vi "get_setting.vi"(7 "settings path":path=path "D:/Scripts/AId_SPM_labview/Nanonis Server", 8 "error in (no error)":errorcluster, 9 "section":string="Settings", 10 "FirstRun":bool, 11 "key":string) -> (0 "error out":errorcluster, 1 "output 2":dbl, 2 "output 1":dbl, 3 "value":string="Loaded from:C:\\Users\\cornelik\\AId_SPM_labview\\Nanonis Server\\AId_SPM_server.ini", 4 "Boolean":bool)   [LabVIEW 2019]
uses:
  <vilib>/Utility/config.llb/Read Key (String).vi
  <vilib>/Utility/config.llb/NI_LVConfig.lvlib
panel:
  out "keys":string[][](array[string])
  out "values":string[][](array[string])
  out "sections":string[](array[string])
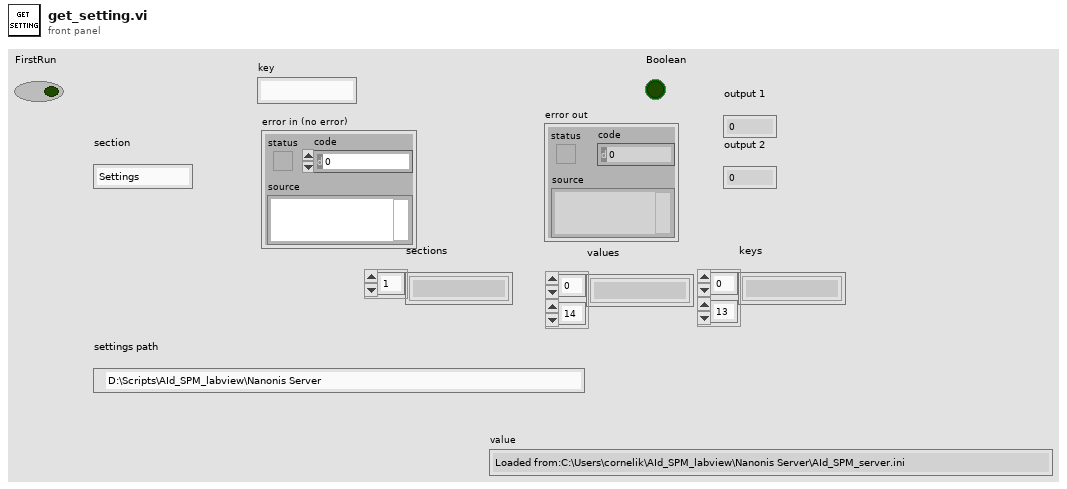
[diagram p1: front panel]
types:
  T1 = typedef "NI_LVConfig.lvlib/Config Data RefNum.ctl" = refnum<k1>
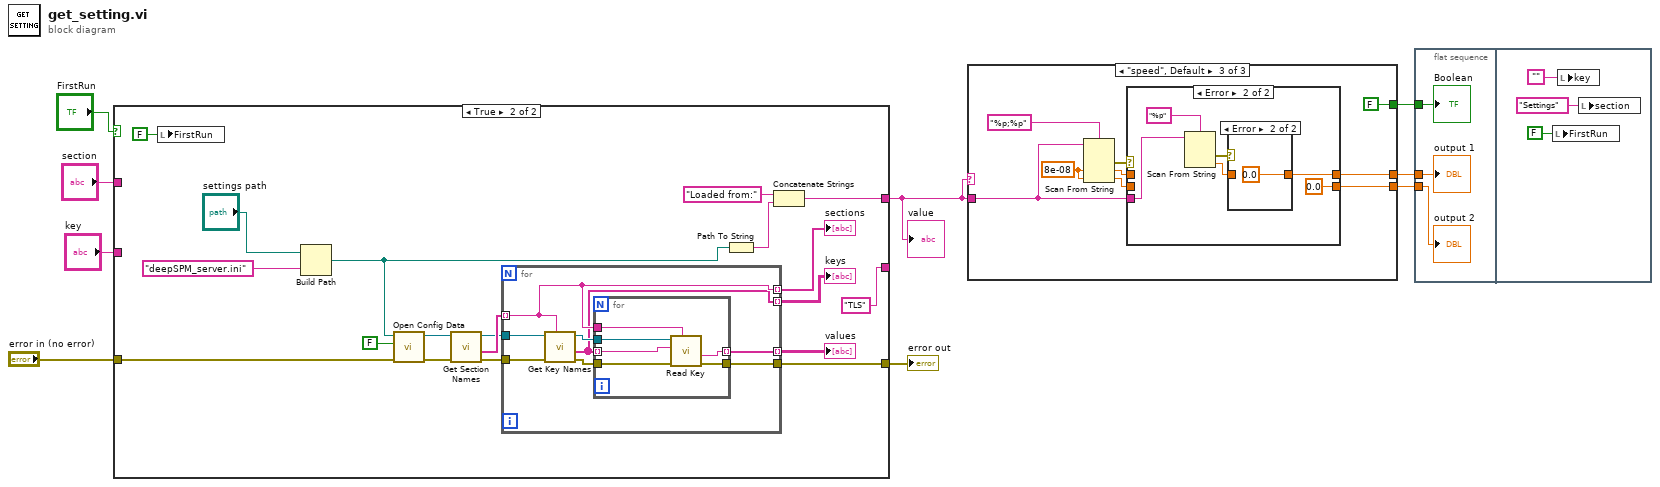
[diagram p0: block diagram]
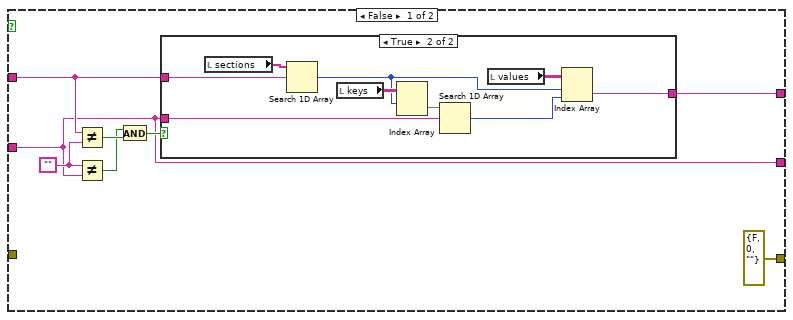
[diagram p2: hidden frame]
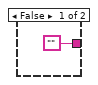
[diagram p3: hidden frame]
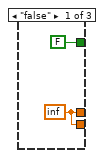
[diagram p4: hidden frame]
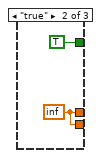
[diagram p5: hidden frame]
diagram:
  n1 = case shown="True" "FirstRun" {
    tunnel: "section" -> [w12 _]
    tunnel: [w17 w32] -> w1
    tunnel: "key" -> [w10 _]
    tunnel: "error in (no error)" -> [_ w35]
    tunnel: [errorcluster {"status"=FALSE, "code"=0, "source"=""} ("error out") w34] -> w4
    tunnel: [w10 "TLS" ("key")] -> _
    frame False {
      w11 = ""
      n2 = Not Equal?(x=w12, y=w11) -> (x != y?=w15:bool)
      n3 = Not Equal?(x=w11, y=w10) -> (x != y?=w13:bool)
      n4 = And(x=w13, y=w15) -> (x .and. y?=w14:bool)
      n5 = case shown="True" w14 {
        tunnel: w12 -> [_ w26]
        tunnel: w10 -> [_ w23]
        tunnel: ["" w20] -> w17
        frame False {
        }
        frame True {
          n6 = local read "sections"() -> (w27:string[])
          n7 = Search 1D Array(1D array=w27, element=w26) -> (index of element=w19:i32)  [unwired: 1 in]
          n8 = local read "keys"() -> (w25:string[][])
          n9 = Index Array(array=w25, index (row)=w19) -> (element=w24:string[])  [unwired: 1 in]
          n10 = Search 1D Array(1D array=w24, element=w23) -> (index of element=w21:i32)  [unwired: 1 in]
          n11 = local read "values"() -> (w22:string[][])
          n12 = Index Array(array=w22, index (row)=w19, index (col)=w21) -> (element=w20:string)
        }
      }
    }
    frame True {
      n13 = local write "FirstRun"(FALSE ("FirstRun")) -> ()
      n14 = Build Path(base path="settings path", name or relative path="deepSPM_server.ini") -> (appended path=w31:path)
      n15 = call <vilib>:"Open Config Data.vi"("error in (no error)"=w35, "create file if necessary (T)"=FALSE, "configuration file path"=w31) -> ("error out"=w43:errorcluster, "refnum"=w44:T1)  [unwired: 6 in, 1 out]
      n16 = call <vilib>:"Get Section Names.vi"("error in (no error)"=w43, "refnum"=w44) -> ("error out"=w40:errorcluster, "section names"=w42:string[], "refnum out"=w41:T1)  [unwired: 7 in]
      n17 = for {
        tunnel: w42 -> [w49] mode=indexing
        tunnel: w41 -> [w52]
        tunnel: w40 -> [w51]
        tunnel: [w50] -> w38 mode=indexing
        tunnel: [w49] -> w39 mode=indexing
        tunnel: [w48] -> w37 mode=indexing
        tunnel: [w47] -> w34
        n18 = call <vilib>:"Get Key Names.vi"("section"=w49, "error in (no error)"=w51, "refnum"=w52) -> ("error out"=w54:errorcluster, "key names"=w48:string[], "refnum out"=w53:T1)  [unwired: 5 in, 1 out]
        n19 = for {
          tunnel: w54 -> [w60]
          tunnel: w53 -> [w59]
          tunnel: w49 -> [w58]
          tunnel: w48 -> [w57] mode=indexing
          tunnel: [w56] -> w50 mode=indexing
          tunnel: [w55] -> w47
          n20 = call-poly <vilib>:"Read Key.vi"("section"=w58, "error in (no error)"=w60, "key"=w57, "refnum"=w59) -> ("error out"=w55:errorcluster, "value"=w56:string)  [unwired: 4 in, 2 out]
        }
      }
      "sections" <- w39
      "values" <- w38
      "keys" <- w37
      n21 = Path To String(path=w31) -> (string=w30:string)
      n22 = Concatenate Strings("Loaded from:" ("value"), w30) -> (w32:string)
    }
  }
  "value" <- w1
  "error out" <- w4
  n23 = case shown="\"speed\", Default" w1 {
    tunnel: w1 -> [_ _ w69]
    tunnel: [w62 w64 w67] -> w2
    tunnel: [w62 w64 w65] -> w3
    tunnel: [FALSE TRUE FALSE] -> w7
    frame "false" {
      w62 = inf
    }
    frame "true" {
      w64 = inf
    }
    frame "speed", Default {
      w71 = 8e-08 ("default value 1")
      n24 = Scan From String(format string="%p;%p", input string=w69, default 1=w71, default 2=w71) -> (error out=w70:errorcluster, output 1=w68:dbl, output 2=w66:dbl)  [unwired: 2 in, 2 out]
      n25 = case shown="Error" w70 {
        tunnel: w69 -> [_ w80]
        tunnel: w68 -> [w75 _]
        tunnel: [w75 w77] -> w67
        tunnel: w66 -> [w74 _]
        tunnel: [w74 0.0 ("default value 1")] -> w65
        frame No Error {
        }
        frame Error {
          n26 = Scan From String(format string="%p", input string=w80) -> (error out=w78:errorcluster, output 1=w76:dbl)  [unwired: 3 in, 2 out]
          n27 = case shown="Error" w78 {
            tunnel: [w82 0.0] -> w77
            tunnel: w76 -> [w82 _]
            frame No Error {
            }
            frame Error {
            }
          }
        }
      }
    }
  }
  n28 = flat-sequence {
    tunnel: w7 -> [w86]
    tunnel: w3 -> [w85]
    tunnel: w2 -> [w84]
    frame #0 {
      "Boolean" <- w86
      "output 1" <- w84
      "output 2" <- w85
    }
    frame #1 {
      n29 = local write "FirstRun"(FALSE ("FirstRun")) -> ()
      n30 = local write "key"("") -> ()
      n31 = local write "section"("Settings" ("section")) -> ()
    }
  }
